vi "host_scan_config.vi"(8 "error in":errorcluster, 11 "scan config":T1) -> (0 "error out":errorcluster)   [LabVIEW 2021]
doc: "Set scan configuration. This vi should be called before start the scan."
uses:
  fpga/fpga_dtype_scan_config.ctl
  fpga/fpga_dtype_sgl_8ch.ctl
  core/host_global_vars.vi
  <vilib>/Utility/error.llb/Error Cluster From Error Code.vi
  <vilib>/rvi/errors/niLvFpgaAdjustHostInterfaceError.vi
  <vilib>/rvi/interface/nirviReadWriteControl/nirviReadWriteControl.xnode
  FPGA Bitfiles/openlabspm_FPGATarget_fpgamain_eo-gUZR5D1g.lvbitx
  fpga/fpga_main.vi
  NiFpgaLv.dll
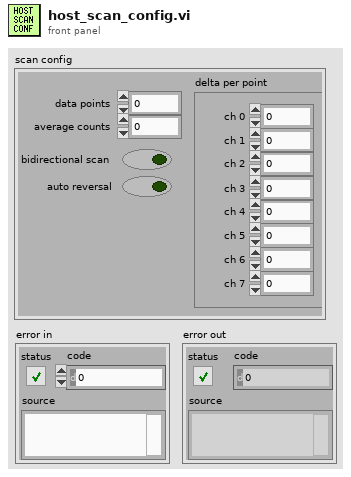
[diagram p1: front panel]
types:
  T1 = typedef "fpga_dtype_scan_config.ctl" = cluster{"data points":i16, "average counts":i16, "delta per point":T2, "bidirectional scan":bool, "auto reversal":bool}
  T2 = typedef "fpga_dtype_sgl_8ch.ctl" = cluster{"ch 0":sgl, "ch 1":sgl, "ch 2":sgl, "ch 3":sgl, "ch 4":sgl, "ch 5":sgl, "ch 6":sgl, "ch 7":sgl}
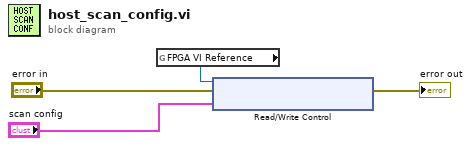
[diagram p0: block diagram]
diagram:
  n1 = global read "host_global_vars.vi" "FPGA VI Reference"() -> (w3:refnum<k20>)
  n2 = xnode "Read/Write Control"("FPGA VI Reference In"=w3, "error in"="error in", "scan config"="scan config") -> ("error out"=→"error out":errorcluster)  [unwired: 1 out]
